vi "Display Calibration Results.vi"(11 "Fit Data":T1(array[cluster])) -> ()   [LabVIEW 2015, in "Calibration UI.lvclass"]
doc: "This is a pop-up window that is displayed when calibrations are complete. The slopes and intercepts as captured by the given SVs will be updated and sent to the server."
uses:
  Calibration UI.lvclass
panel:
  in  "end":bool
  in  "Calibration Data":T2 {"r^2"."Cell 5" format="%.2f"; "r^2"."Cell 4" format="%.2f"; "r^2"."Cell 3" format="%.2f"; "r^2"."Cell 2" format="%.2f"; "r^2"."Cell 1" format="%.2f"; "Intercepts"."Cell 5" format="%.2e"; "Intercepts"."Cell 4" format="%.2e"; "Intercepts"."Cell 3" format="%.2e"; "Intercepts"."Cell 2" format="%.2e"; "Intercepts"."Cell 1" format="%.2e"; "Slopes"."Cell 5" format="%.2e"; "Slopes"."Cell 4" format="%.2e"; "Slopes"."Cell 3" format="%.2e"; "Slopes"."Cell 2" format="%.2e"; "Slopes"."Cell 1" format="%.2e"}
  # "TD  - 660"
  # "Dry - 532"
  # "Dry  - 660"
  # "Dry  - 405"
  # "TD - 405"
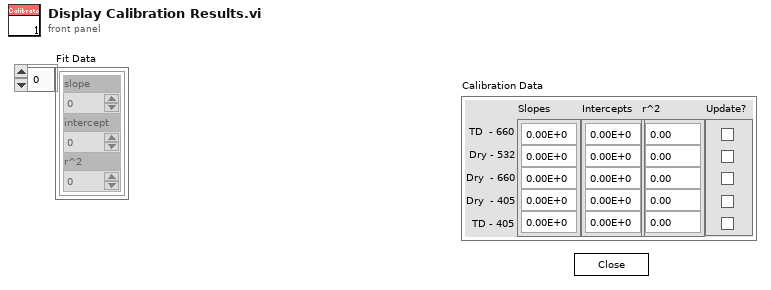
[diagram p1: front panel]
types:
  T1 = cluster{"slope":dbl, "intercept":dbl, "r^2":dbl}[]
  T2 = cluster{"Slopes":cluster{"Cell 1":sgl, "Cell 2":sgl, "Cell 3":sgl, "Cell 4":sgl, "Cell 5":sgl}, "Intercepts":cluster{"Cell 1":sgl, "Cell 2":sgl, "Cell 3":sgl, "Cell 4":sgl, "Cell 5":sgl}, "r^2":cluster{"Cell 1":sgl, "Cell 2":sgl, "Cell 3":sgl, "Cell 4":sgl, "Cell 5":sgl}, "Update?":cluster{"Cell 1":bool, "Cell 2":bool, "Cell 3":bool, "Cell 4":bool, "Cell 5":bool}}
  T3 = cluster{"[0]":dbl, "[1]":dbl, "[2]":dbl, "[3]":dbl, "[4]":dbl}
  T4 = cluster{"Cell 1":sgl, "Cell 2":sgl, "Cell 3":sgl, "Cell 4":sgl, "Cell 5":sgl}
  T5 = cluster{"Cell 1":bool, "Cell 2":bool, "Cell 3":bool, "Cell 4":bool, "Cell 5":bool}
  T6 = enum32{"Invalid", "Standard", "Closed", "Hidden", "Minimized", "Maximized"}
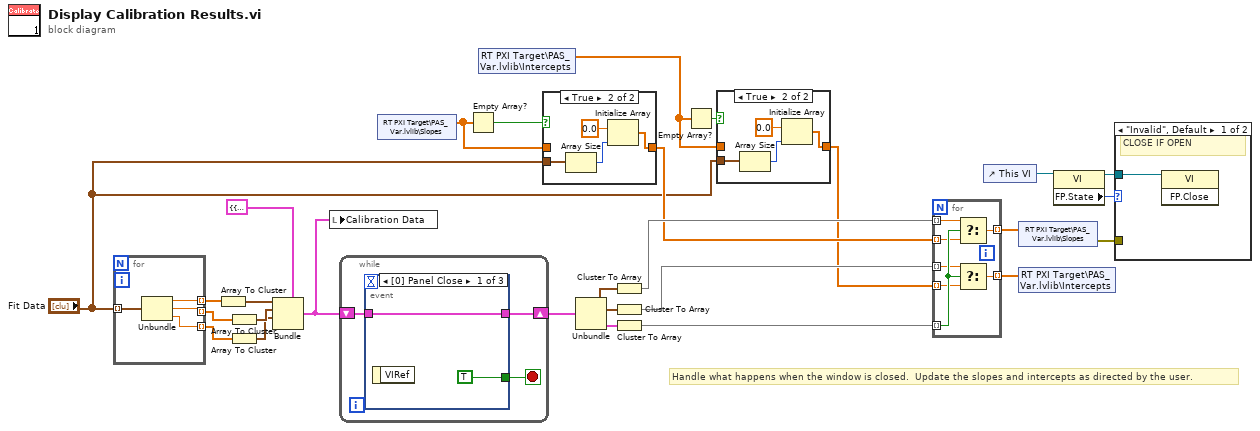
[diagram p0: block diagram]
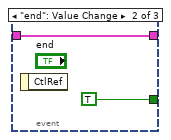
[diagram p5: hidden frame]
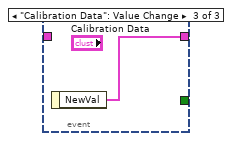
[diagram p6: hidden frame]
diagram:
  # "Handle what happens when the window is closed.  Update the slopes and intercepts as directed by the user."
  n1 = for {
    tunnel: "Fit Data" -> [w32] mode=indexing
    tunnel: [w31] -> w26 mode=indexing
    tunnel: [w30] -> w25 mode=indexing
    tunnel: [w29] -> w11 mode=indexing
    n2 = Unbundle(w32) -> ("slope"=w31:dbl, "intercept"=w30:dbl, "r^2"=w29:dbl)
  }
  n3 = Array To Cluster(array=w26) -> (cluster=w27:T3)
  n4 = Array To Cluster(array=w25) -> (cluster=w28:T3)
  n5 = Array To Cluster(array=w11) -> (cluster=w10:T3)
  n6 = Bundle(cluster=T2 {"Slopes"={"Cell 1"=0.0, "Cell 2"=0.0, "Cell 3"=0.0, "Cell 4"=0.0, "Cell 5"=0.0}, "Intercepts"={"Cell 1"=0.0, "Cell 2"=0.0, "Cell 3"=0.0, "Cell 4"=0.0, "Cell 5"=0.0}, "r^2"={"Cell 1"=0.0, "Cell 2"=0.0, "Cell 3"=0.0, "Cell 4"=0.0, "Cell 5"=0.0}, "Update?"={"Cell 1"=FALSE, "Cell 2"=FALSE, "Cell 3"=FALSE, "Cell 4"=FALSE, "Cell 5"=FALSE}} ("Calibration Data"), "Slopes"=w27, "Intercepts"=w28, "r^2"=w10) -> (w9:T2)  [unwired: 1 in]
  n7 = local write "Calibration Data"(w9) -> ()
  n8 = while {
    shift-right: [w33] -> w2
    shift-left: w9 -> [w34]
    stop <- w35 stop-if-true
    n9 = event shown="[0] Panel Close" {
      selector: _ -> [_ _ _]
      dyn-events: _ -> [_ _ _]
      timeout: _ -> [_ _ _]
      tunnel: [TRUE TRUE _] -> w35
      tunnel: w34 -> [w36 w38 _]
      tunnel: [w36 w38 w40] -> w33
      event Panel Close {
        n10 = event-data() -> ()  [unwired: 1 in, 1 out]
      }
      event "end": Value Change {
        n11 = event-data() -> ()  [unwired: 1 in, 1 out]
      }
      event "Calibration Data": Value Change {
        n12 = event-data() -> ("NewVal"=w40:T2)  [unwired: 1 in]
      }
    }
  }
  n13 = shared-variable "RT PXI Target\\PAS_Var.lvlib\\Slopes"() -> (w7:sgl[])  [unwired: 1 in, 1 out]
  n14 = Empty Array?(array=w7) -> (empty?=w8:bool)
  n15 = shared-variable "RT PXI Target\\PAS_Var.lvlib\\Intercepts"() -> (w4:sgl[])  [unwired: 1 in, 1 out]
  n16 = case shown="True" w8 {
    tunnel: "Fit Data" -> [_ w45]
    tunnel: w7 -> [w41 _]
    tunnel: [w41 w42] -> w6
    frame False {
    }
    frame True {
      n17 = Array Size(array=w45) -> (size(s)=w44:i32)
      n18 = Initialize Array(sgl 0.0 ("element"), w44) -> (w42:sgl[])
    }
  }
  n19 = Unbundle(w2) -> ("Slopes"=w17:T4, "Intercepts"=w18:T4, "Update?"=w20:T5)  [unwired: 1 out]
  n20 = Cluster To Array(cluster=w17) -> (array=w16:sgl[])
  n21 = Cluster To Array(cluster=w18) -> (array=w14:sgl[])
  n22 = Cluster To Array(cluster=w20) -> (array=w19:bool[])
  n23 = Empty Array?(array=w4) -> (empty?=w5:bool)
  n24 = case shown="True" w5 {
    tunnel: "Fit Data" -> [_ w50]
    tunnel: w4 -> [w46 _]
    tunnel: [w46 w47] -> w3
    frame False {
    }
    frame True {
      n25 = Array Size(array=w50) -> (size(s)=w49:i32)
      n26 = Initialize Array(sgl 0.0 ("element"), w49) -> (w47:sgl[])
    }
  }
  n27 = for {
    tunnel: w19 -> [w57] mode=indexing
    tunnel: w16 -> [w56] mode=indexing
    tunnel: w6 -> [w55] mode=indexing
    tunnel: [w54] -> w15 mode=indexing
    tunnel: w14 -> [w53] mode=indexing
    tunnel: w3 -> [w52] mode=indexing
    tunnel: [w51] -> w13 mode=indexing
    n28 = Select(t=w56, s=w57, f=w55) -> (s? t:f=w54:sgl)
    n29 = Select(t=w53, s=w57, f=w52) -> (s? t:f=w51:sgl)
  }
  n30 = control-ref of="This VI"() -> (w24:refnum<vi>)
  n31 = shared-variable "RT PXI Target\\PAS_Var.lvlib\\Slopes"(w15) -> (error out=w12:errorcluster)  [unwired: 1 in]
  n32 = shared-variable "RT PXI Target\\PAS_Var.lvlib\\Intercepts"(w13) -> ()  [unwired: 1 in, 1 out]
  n33 = property class="VI"(reference=w24) -> (reference out=w22:refnum<vi>, "FP.State"=w23:T6)  [unwired: 1 in, 1 out]
  n34 = case shown="\"Invalid\", Default" w23 {
    tunnel: w22 -> [w58 _]
    tunnel: w12 -> [_ _]
    frame "Invalid", Default {
      # "CLOSE IF OPEN"
      n35 = invoke class="VI" method="FP.Close"(reference=w58) -> ()  [unwired: 2 in, 3 out]
    }
    frame "Closed" {
    }
  }
